vi "Scale A B Mode.vi"(0 "VISA resource name":refnum<visa-resource-name>, 1 "Maximum A (1.0E+6)":dbl=1000000.0 min=-9.999e+37 max=9.99e+37 format="%^.3e", 2 "Minimum A (0.0)":dbl min=-9.999e+37 max=1e+38 format="%^.3e", 5 "Scale Division A (5.0E-3)":dbl=0.005 min=5e-36 max=9.999e+36 format="%^.3e", 7 "Scale (0:Autoscale A/B)":u32(ring) items=["Autoscale  A/B", "Min/Max A", "Min/Max B", "Scale Division A", "Scale Division B"], 9 "Minimum B (0.0)":dbl min=-1e+38 max=9.99e+37 format="%^.3e", 11 "error in (no error)":errorcluster, 12 "Maximum B (1.0E+6)":dbl=1000000.0 min=-9.999e+37 max=9.99e+37 format="%^.3e", 13 "Scale Division B (5.0E-3)":dbl=0.005 min=5e-36 max=9.999e+36 format="%^.3e") -> (4 "VISA resource name out":refnum<visa-resource-name>, 15 "error out":errorcluster)   [LabVIEW 2010, in "Agilent 4194.lvlib"]
doc: "This function sets the display scale parameters effective for A-B.\n\nNotes:\n\n(1) This function is valid for A-B setting only."
uses:
  <instrlib>/Agilent 4194/Agilent 4194.lvlib
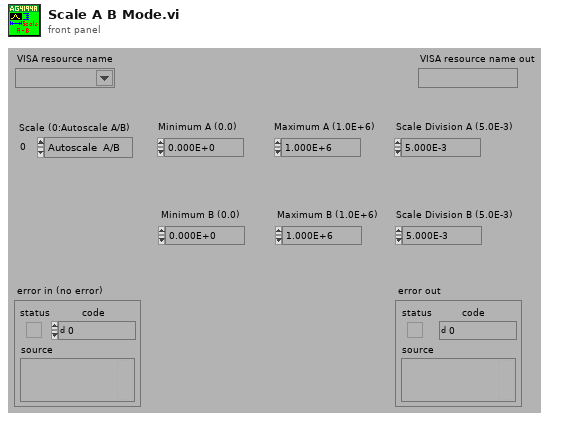
[diagram p1: front panel]
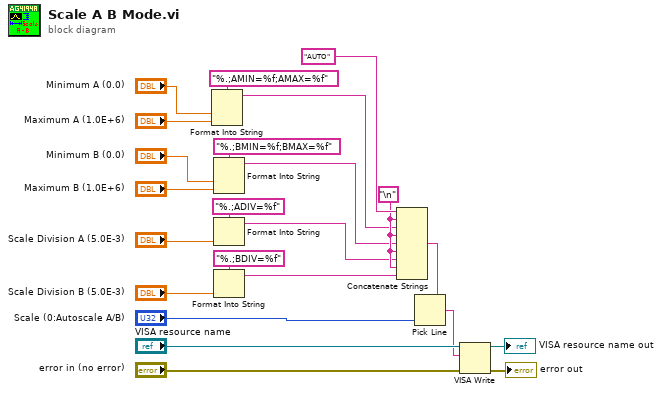
[diagram p0: block diagram]
diagram:
  w5 = "\n"
  n1 = Format Into String(format string="%.;AMIN=%f;AMAX=%f", "Minimum A (0.0)", "Maximum A (1.0E+6)") -> (resulting string=w4:string)  [unwired: 2 in, 1 out]
  n2 = Format Into String(format string="%.;BMIN=%f;BMAX=%f", "Minimum B (0.0)", "Maximum B (1.0E+6)") -> (resulting string=w3:string)  [unwired: 2 in, 1 out]
  n3 = Format Into String(format string="%.;ADIV=%f", "Scale Division A (5.0E-3)") -> (resulting string=w2:string)  [unwired: 2 in, 1 out]
  n4 = Format Into String(format string="%.;BDIV=%f", "Scale Division B (5.0E-3)") -> (resulting string=w1:string)  [unwired: 2 in, 1 out]
  n5 = Concatenate Strings("AUTO", w5, w4, w5, w3, w5, w2, w5, w1) -> (w18:string)
  n6 = Pick Line(multi-line string=w18, line index="Scale (0:Autoscale A/B)") -> (output string=w7:string)  [unwired: 1 in]
  n7 = VISA Write(VISA resource name="VISA resource name", write buffer=w7, error in (no error)="error in (no error)") -> (VISA resource name out=→"VISA resource name out":refnum<visa-resource-name>, error out=→"error out":errorcluster)  [unwired: 1 out]
